vi "Start Calculation.vi"(8 "error in (no error)":errorcluster, 10 "appended array":T1[](array[typedef]) {"Zoom Parameters"."fwidth:" format="%#_6p"; "Zoom Parameters"."f0:" format="%#_6p"}, 11 "GPU FFT Calculator in":refnum<class "GPU FFT Calculator.lvclass">) -> (0 "error out":errorcluster, 3 "GPU FFT Calculator out":refnum<class "GPU FFT Calculator.lvclass">)   [LabVIEW 2020, in "GPU FFT Calculator.lvlib" / "GPU FFT Calculator.lvclass"]
uses:
  GPU FFT Calculator.lvclass
  C:/Users/natan/Documents/G2CPU-Performance-Demo/Calculation Worker/Calculation Worker/Calculation Worker.lvclass
  C:/Program Files/National Instruments/LabVIEW 2026/vi.lib/ActorFramework/Actor/Actor.lvclass
  GPU Calculation Message.ctl
  <vilib>/Natan Biesmans/G2CPU GPU and CPU HPC Toolkit/G2CPU Libraries/Async IO/DMA Manager/DMA Manager.lvclass
  <vilib>/Natan Biesmans/G2CPU GPU and CPU HPC Toolkit/G2CPU Libraries/Arrays/1DArray/s16/1D Array s16.lvclass
  <vilib>/Natan Biesmans/G2CPU GPU and CPU HPC Toolkit/G2CPU Libraries/Arrays/1DArray/f32/1D Array f32.lvclass
  chart zoom.ctl
  GPU Metrics.ctl
  <vilib>/ActorFramework/Actor/Actor.lvclass/Actor.ctl
  <vilib>/ActorFramework/Message Enqueuer/Message Enqueuer.lvclass/Message Enqueuer.ctl
  GPU FFT Calculator Messages/Do Calculation Msg/Do Calculation Msg.lvclass/Do Calculation Msg.ctl
  Application Manager/Application Manager Messages/Set UI GPU Done Msg/Set UI GPU Done Msg.lvclass/Set UI GPU Done Msg.ctl
  <vilib>/ActorFramework/Message Enqueuer/Init from Existing Queue.vi
  <vilib>/ActorFramework/Message Enqueuer/Enqueue.vi
  GPU FFT Calculator Messages/Do Calculation Msg/Do Calculation Msg.lvclass
  C:/Program Files/National Instruments/LabVIEW 2026/vi.lib/ActorFramework/Message/Message.lvclass
  Application Manager/Application Manager Messages/Set UI GPU Done Msg/Set UI GPU Done Msg.lvclass
  <vilib>/ActorFramework/Message Priority Queue/Priority Enqueue.vi
  <vilib>/ActorFramework/Message Enqueuer/Message Enqueuer.lvclass
  <vilib>/ActorFramework/Actor/Actor.lvclass
  Simple UI/Simple UI/Simple UI.lvclass
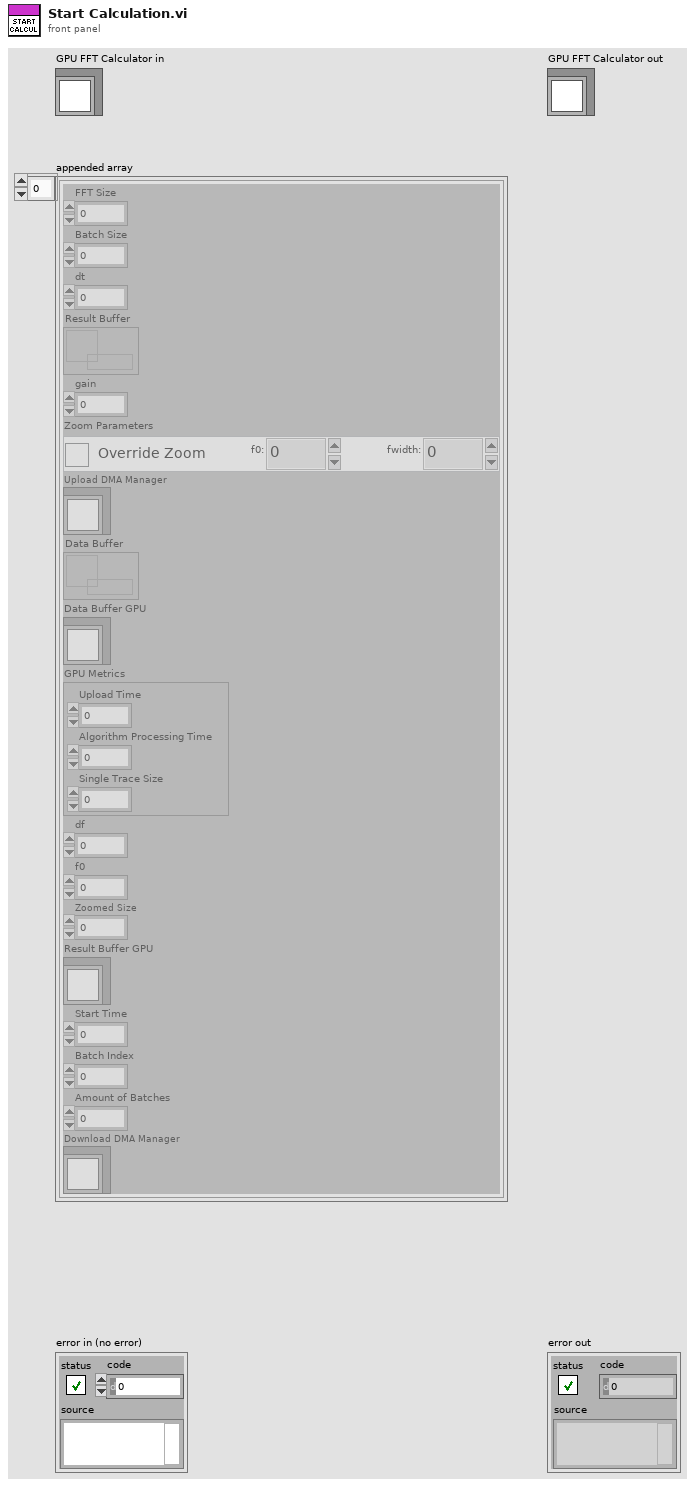
[diagram p1: front panel]
types:
  T1 = typedef "GPU FFT Calculator.lvlib/GPU FFT Calculator.lvclass/GPU Calculation Message.ctl" = cluster{"FFT Size":u64, "Batch Size":u64, "dt":dbl, "Result Buffer":refnum<data-value>, "gain":dbl, "Zoom Parameters":T2, "Upload DMA Manager":refnum<class "DMA Manager.lvclass">, "Data Buffer":refnum<data-value>, "Data Buffer GPU":refnum<class "1D Array s16.lvclass">, "GPU Metrics":T3, "df":dbl, "f0":dbl, "Zoomed Size":u64, "Result Buffer GPU":refnum<class "1D Array f32.lvclass">, "Start Time":dbl, "Batch Index":i32, "Amount of Batches":i32, "Download DMA Manager":refnum<class "DMA Manager.lvclass">}
  T2 = typedef "Simple UI.lvlib/Simple UI.lvclass/chart zoom.ctl" = cluster{"Override":bool, "f0: ":dbl, "fwidth: ":dbl}
  T3 = typedef "GPU FFT Calculator.lvlib/GPU FFT Calculator.lvclass/GPU Metrics.ctl" = cluster{"Upload Time":dbl, "Algorithm Processing Time":dbl, "Single Trace Size":u64}
  T4 = typedef "Data Source.lvlib/Data Source.lvclass/Data Source Buffer.ctl" = refnum<data-value>
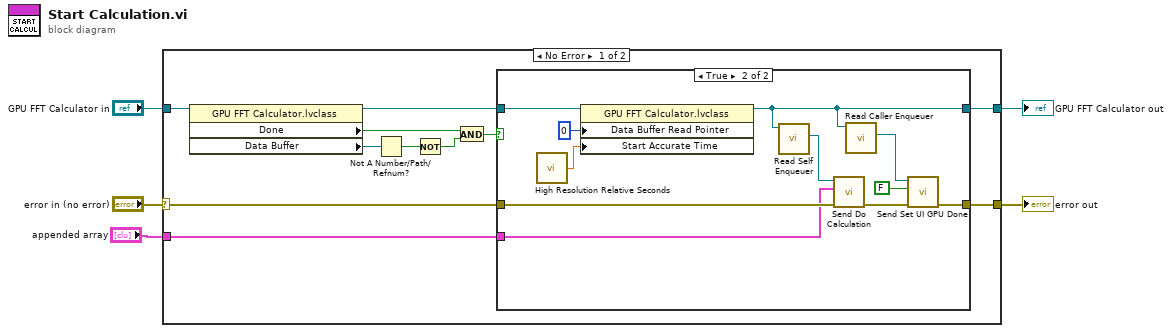
[diagram p0: block diagram]
diagram:
  n1 = case shown="No Error" "error in (no error)" {
    selector: "error in (no error)" -> [w15 w31]
    tunnel: [w13 w31] -> w4
    tunnel: [w14 w30] -> w2
    tunnel: "GPU FFT Calculator in" -> [w16 w30]
    tunnel: "appended array" -> [w6 _]
    frame No Error {
      n2 = property class="GPU FFT Calculator.lvclass"(reference=w16) -> (reference out=w12:refnum<class "GPU FFT Calculator.lvclass">, "Done"=w9:bool, "Data Buffer"=w8:T4)  [unwired: 1 in, 1 out]
      n3 = Not A Number/Path/Refnum?(number/path/refnum=w8) -> (NaN/Path/Refnum?=w11:bool)
      n4 = Not(x=w11) -> (.not. x?=w10:bool)
      n5 = And(x=w9, y=w10) -> (x .and. y?=w7:bool)
      n6 = case shown="True" w7 {
        tunnel: w15 -> [w17 w28]
        tunnel: [w18 w26] -> w14
        tunnel: [w17 w23] -> w13
        tunnel: w12 -> [w18 w20]
        tunnel: w6 -> [_ w19]
        frame False {
        }
        frame True {
          n7 = call <vilib>:"High Resolution Relative Seconds.vi"() -> ("relative seconds"=w21:dbl)
          n8 = property class="GPU FFT Calculator.lvclass"(reference=w20, "Data Buffer Read Pointer"=u64 0, "Start Accurate Time"=w21) -> (reference out=w26:refnum<class "GPU FFT Calculator.lvclass">)  [unwired: 1 in, 1 out]
          n9 = call <vilib>:"Read Self Enqueuer.vi"("Actor"=w26) -> ("Self Enqueuer"=w27:refnum<class "Message Enqueuer.lvclass">)  [unwired: 10 in]
          n10 = call "Send Do Calculation.vi"("error in (no error)"=w28, "Array"=w19, "Message Enqueuer"=w27) -> ("error out"=w25:errorcluster)  [unwired: 7 in, 1 out]
          n11 = call <vilib>:"Read Caller Enqueuer.vi"("Actor"=w26) -> ("Caller Enqueuer"=w24:refnum<class "Message Enqueuer.lvclass">)  [unwired: 10 in]
          n12 = call "Send Set UI GPU Done.vi"("error in (no error)"=w25, "GPU Done"=FALSE, "Message Enqueuer"=w24) -> ("error out"=w23:errorcluster)  [unwired: 7 in, 1 out]
        }
      }
    }
    frame Error {
    }
  }
  "error out" <- w4
  "GPU FFT Calculator out" <- w2
